vi "sub_pf_observation.vi"(8 "rf_id":cluster{"x":dbl, "y":dbl}[](array[cluster]), 9 "u":T1, 10 "xd":T1, 11 "x_true":T1) -> (0 "ud":T1, 1 "xd out":T1, 2 "z":T1, 3 "x_true out":T1)   [LabVIEW 2019]
uses:
  <vilib>/Analysis/Matrix/Datatypes/RealMatrix.ctl
  Ctrl/cmd_common.ctl
  <vilib>/ptbypt/NI_PtbyPt.lvlib
  <vilib>/Analysis/Matrix/NI_Matrix.lvlib
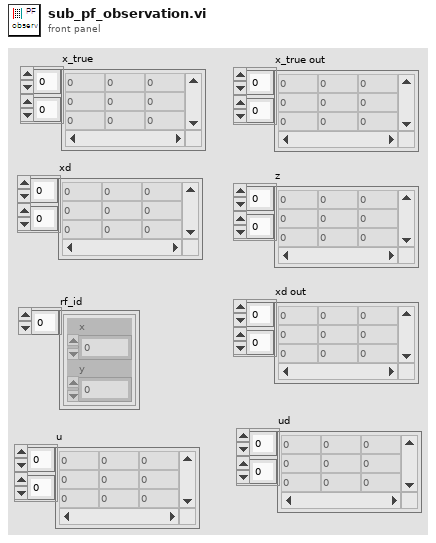
[diagram p1: front panel]
types:
  T1 = typedef "NI_Matrix.lvlib/RealMatrix.ctl" = dbl[][]
  T2 = typedef "cmd_common.ctl" = enum16{"read", "write"}
  T3 = cluster{"DT":dbl, "SIM_TIME":dbl, "MAX_RANGE":dbl, "NP":u32, "NTh":u32, "Q":T1, "R":T1, "Q_sim":T1, "R_sim":T1, "rf_id":cluster{"x":dbl, "y":dbl}[]}
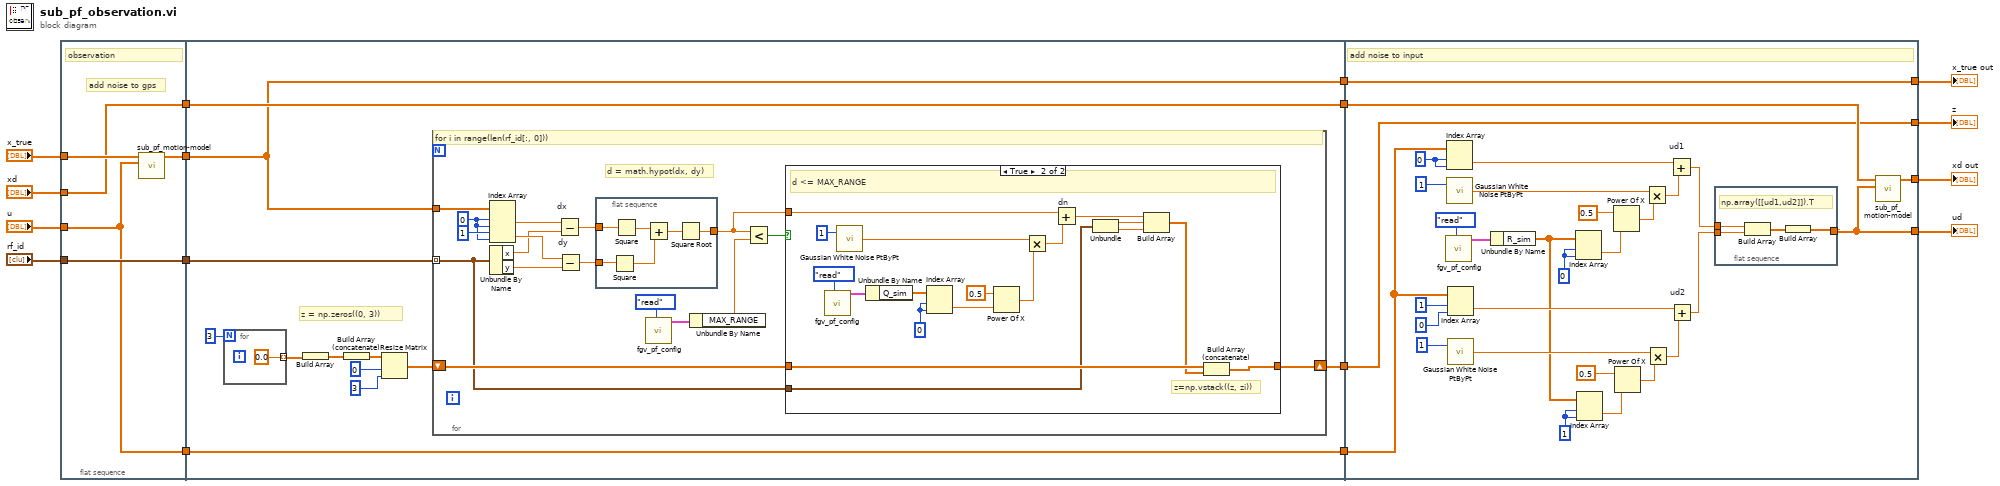
[diagram p0: block diagram]
diagram:
  n1 = flat-sequence {
    tunnel: "u" -> [w18]
    tunnel: [w21] -> w16
    tunnel: "x_true" -> [w19]
    tunnel: "rf_id" -> [w21]
    tunnel: [w17] -> w15
    tunnel: [w18] -> w14
    tunnel: [w20] -> w13
    tunnel: "xd" -> [w17]
    tunnel: w16 -> [w22]
    tunnel: [w31] -> w12
    tunnel: [w33] -> w11
    tunnel: w15 -> [w32]
    tunnel: [w32] -> w10
    tunnel: [w30] -> w9
    tunnel: w14 -> [w31]
    tunnel: w13 -> [w30]
    tunnel: w12 -> [w85]
    tunnel: [w82] -> w2
    tunnel: [w81] -> w3
    tunnel: w11 -> [w78]
    tunnel: [w78] -> w4
    tunnel: w10 -> [w80]
    tunnel: w9 -> [w79]
    tunnel: [w79] -> w6
    frame #0 {
      # "add noise to gps"
      # "observation"
      n2 = call "sub_pf_motion-model.vi"("u"=w18, "x_true"=w19) -> ("x_true out"=w20:T1)  [unwired: 9 in]
    }
    frame #1 {
      # "z = np.zeros((0, 3))"
      n3 = for {
        N: 3 -> [_]
        tunnel: [0.0] -> w28 mode=indexing
      }
      n4 = Build Array(w28) -> (w27:dbl[][])
      n5 = Build Array (concatenate)(w27) -> (w26:T1)
      n6 = Resize Matrix(1:3 ("행의 개수"), 2:0 ("행의 개수"), 4:w26) -> (0:w25:T1)
      n7 = for {
        shift-right: [w40] -> w33
        shift-left: w25 -> [w41]
        tunnel: w30 -> [w39]
        tunnel: w22 -> [w35] mode=indexing
        w50 = 0 ("인덱스 (행)")
        # "d = math.hypot(dx, dy)"
        # "for i in range(len(rf_id[:, 0]))"
        n8 = Index Array(array=w39, index (row) #1=w50, index (col) #1=w50, index (row) #2=1 ("인덱스 (행)"), index (col) #2=w50) -> (element #1=w49:dbl, element #2=w48:dbl)
        n9 = Unbundle By Name(w35) -> ("x"=w37:dbl, "y"=w36:dbl)
        n10 = Subtract "dx"(x=w49, y=w37) -> (x-y=w46:dbl)
        n11 = Subtract "dy"(x=w48, y=w36) -> (x-y=w47:dbl)
        n12 = flat-sequence {
          tunnel: w47 -> [w57]
          tunnel: w46 -> [w56]
          tunnel: [w52] -> w38
          frame #0 {
            n13 = Square(x=w57) -> (x^2=w53:dbl)
            n14 = Square(x=w56) -> (x^2=w54:dbl)
            n15 = Add(x=w54, y=w53) -> (x+y=w55:dbl)
            n16 = Square Root(x=w55) -> (sqrt(x)=w52:dbl)
          }
        }
        n17 = call "fgv_pf_config.vi"("cmd"=cmd_common."read") -> ("pf-val out"=w44:T3)  [unwired: 10 in]
        n18 = Unbundle By Name(w44) -> ("MAX_RANGE"=w43:dbl)
        n19 = Less?(x=w38, y=w43) -> (x < y?=w42:bool)
        n20 = case shown="True" w42 {
          tunnel: w38 -> [_ w66]
          tunnel: w41 -> [w58 w61]
          tunnel: [w58 w62] -> w40
          tunnel: w35 -> [_ w59]
          frame False {
          }
          frame True {
            w72 = 0 ("인덱스 (행)")
            # "z=np.vstack((z, zi))"
            # "d <= MAX_RANGE"
            n21 = call "fgv_pf_config.vi"("cmd"=cmd_common."read") -> ("pf-val out"=w74:T3)  [unwired: 10 in]
            n22 = call <vilib>:"Gaussian White Noise PtByPt.vi"("standard deviation"=1 ("samples")) -> ("Gaussian white noise"=w68:dbl)  [unwired: 2 in]
            n23 = Unbundle By Name(w74) -> ("Q_sim"=w73:T1)
            n24 = Index Array(array=w73, index (row)=w72, index (col)=w72) -> (element=w71:dbl)
            n25 = Power Of X(1:w71, 2:0.5 ("y")) -> (0:w69:dbl)
            n26 = Multiply(x=w68, y=w69) -> (x*y=w67:dbl)
            n27 = Add "dn"(x=w66, y=w67) -> (x+y=w65:dbl)
            n28 = Unbundle(w59) -> ("x"=w64:dbl, "y"=w63:dbl)
            n29 = Build Array(w65, w64, w63) -> (w60:T1)
            n30 = Build Array (concatenate)(w61, w60) -> (w62:T1)
          }
        }
      }
    }
    frame #2 {
      w89 = 1 ("인덱스 (행)")
      w102 = 0 ("인덱스 (행)")
      w106 = 0 ("인덱스 (행)")
      # "add noise to input"
      n31 = call "fgv_pf_config.vi"("cmd"=cmd_common."read") -> ("pf-val out"=w103:T3)  [unwired: 10 in]
      n32 = Index Array(array=w85, index (row)=w106, index (col)=w106) -> (element=w96:dbl)
      n33 = call <vilib>:"Gaussian White Noise PtByPt.vi"("standard deviation"=1 ("samples")) -> ("Gaussian white noise"=w97:dbl)  [unwired: 2 in]
      n34 = Index Array(array=w85, index (row)=1 ("인덱스 (행)"), index (col)=0 ("인덱스 (행)")) -> (element=w95:dbl)
      n35 = call <vilib>:"Gaussian White Noise PtByPt.vi"("standard deviation"=1 ("samples")) -> ("Gaussian white noise"=w94:dbl)  [unwired: 2 in]
      n36 = Unbundle By Name(w103) -> ("R_sim"=w77:T1)
      n37 = Index Array(array=w77, index (row)=w102, index (col)=w102) -> (element=w99:dbl)
      n38 = Index Array(array=w77, index (row)=w89, index (col)=w89) -> (element=w92:dbl)
      n39 = Power Of X(1:w99, 2:0.5 ("y")) -> (0:w100:dbl)
      n40 = Power Of X(1:w92, 2:0.5 ("y")) -> (0:w91:dbl)
      n41 = Multiply(x=w97, y=w100) -> (x*y=w98:dbl)
      n42 = Multiply(x=w94, y=w91) -> (x*y=w93:dbl)
      n43 = Add "ud1"(x=w96, y=w98) -> (x+y=w84:dbl)
      n44 = Add "ud2"(x=w95, y=w93) -> (x+y=w83:dbl)
      n45 = flat-sequence {
        tunnel: w84 -> [w110]
        tunnel: w83 -> [w109]
        tunnel: [w108] -> w81
        frame #0 {
          # "np.array([[ud1,ud2]]).T"
          n46 = Build Array(w110, w109) -> (w107:dbl[])
          n47 = Build Array(w107) -> (w108:T1)
        }
      }
      n48 = call "sub_pf_motion-model.vi"("u"=w81, "x_true"=w80) -> ("x_true out"=w82:T1)  [unwired: 9 in]
    }
  }
  "x_true out" <- w6
  "z" <- w4
  "ud" <- w3
  "xd out" <- w2
